vi "APLUS IEC 2015 Setup.vi"(0 "Remote IP Address":string="192.168.1.101", 1 "Instrument":string, 3 "Sample Rate (1: 0.25s)":u16(ring)=1 items=["0.1s", "0.25s", "0.5s", "1s", "2s", "5s"], 5 "Remote Port":u16=502, 7 "V Range (6: 600V)":u16(ring) items=["Auto", "15V", "30V", "60V", "150V", "300V", "600V"], 9 "A Range (12: 20A)":u16(ring) items=["Auto", "5mA", "10mA", "20mA", "50mA", "100mA", "200mA", "0.5A", "1A", "2A", "5A", "10A", "20A", "50mV", "100mV", "200mV", "2.5V", "5V", "10V"], 11 "error in":errorcluster, 13 "Reset WattHours":bool) -> (2 "VTHD":sgl format="%.3g", 6 "Header File":string[][](array[string]), 15 "error out":errorcluster)   [LabVIEW 2020]
uses:
  Type Definitions/APLUS Commands.ctl
  <vilib>/NI/Modbus Library/API/Wrapper/Create TCP Master.vi
  <vilib>/NI/Modbus Library/API/Master/Modbus Master.lvclass
  <vilib>/NI/Modbus Library/API/Wrapper/API Main.lvlib
panel:
  out "Date & Time":string
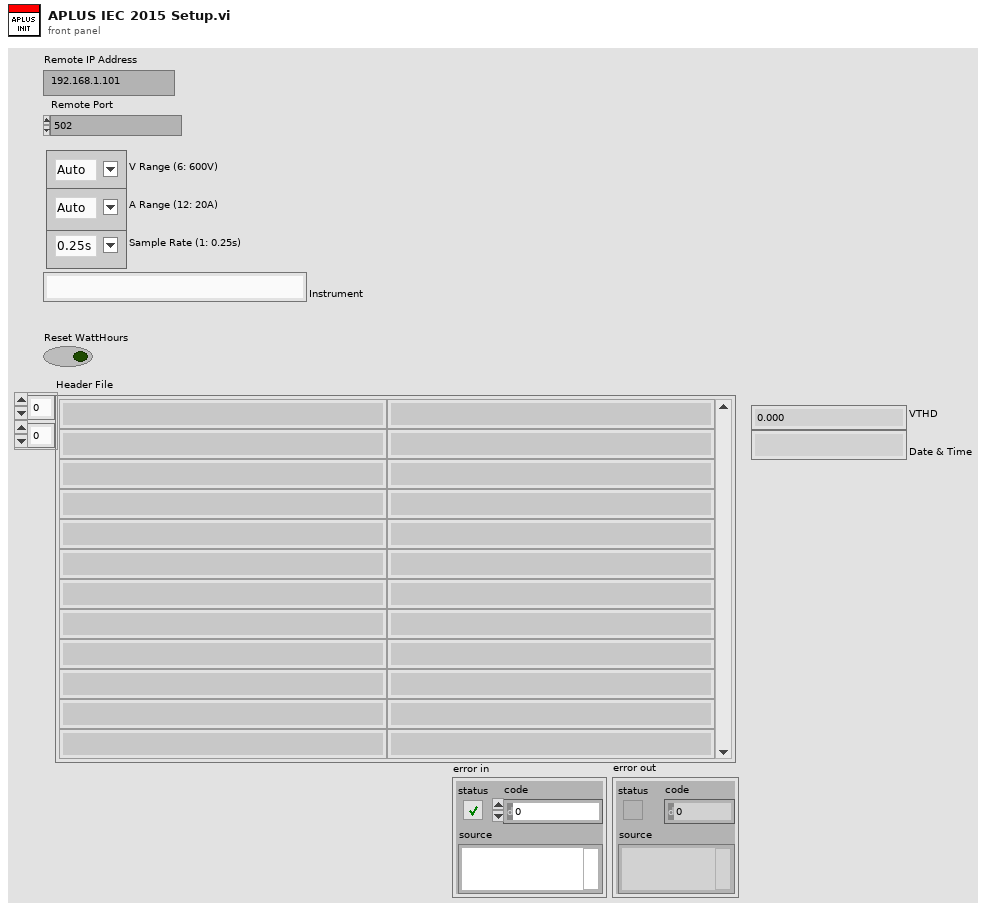
[diagram p1: front panel]
types:
  T1 = typedef "APLUS Commands.ctl" = u16
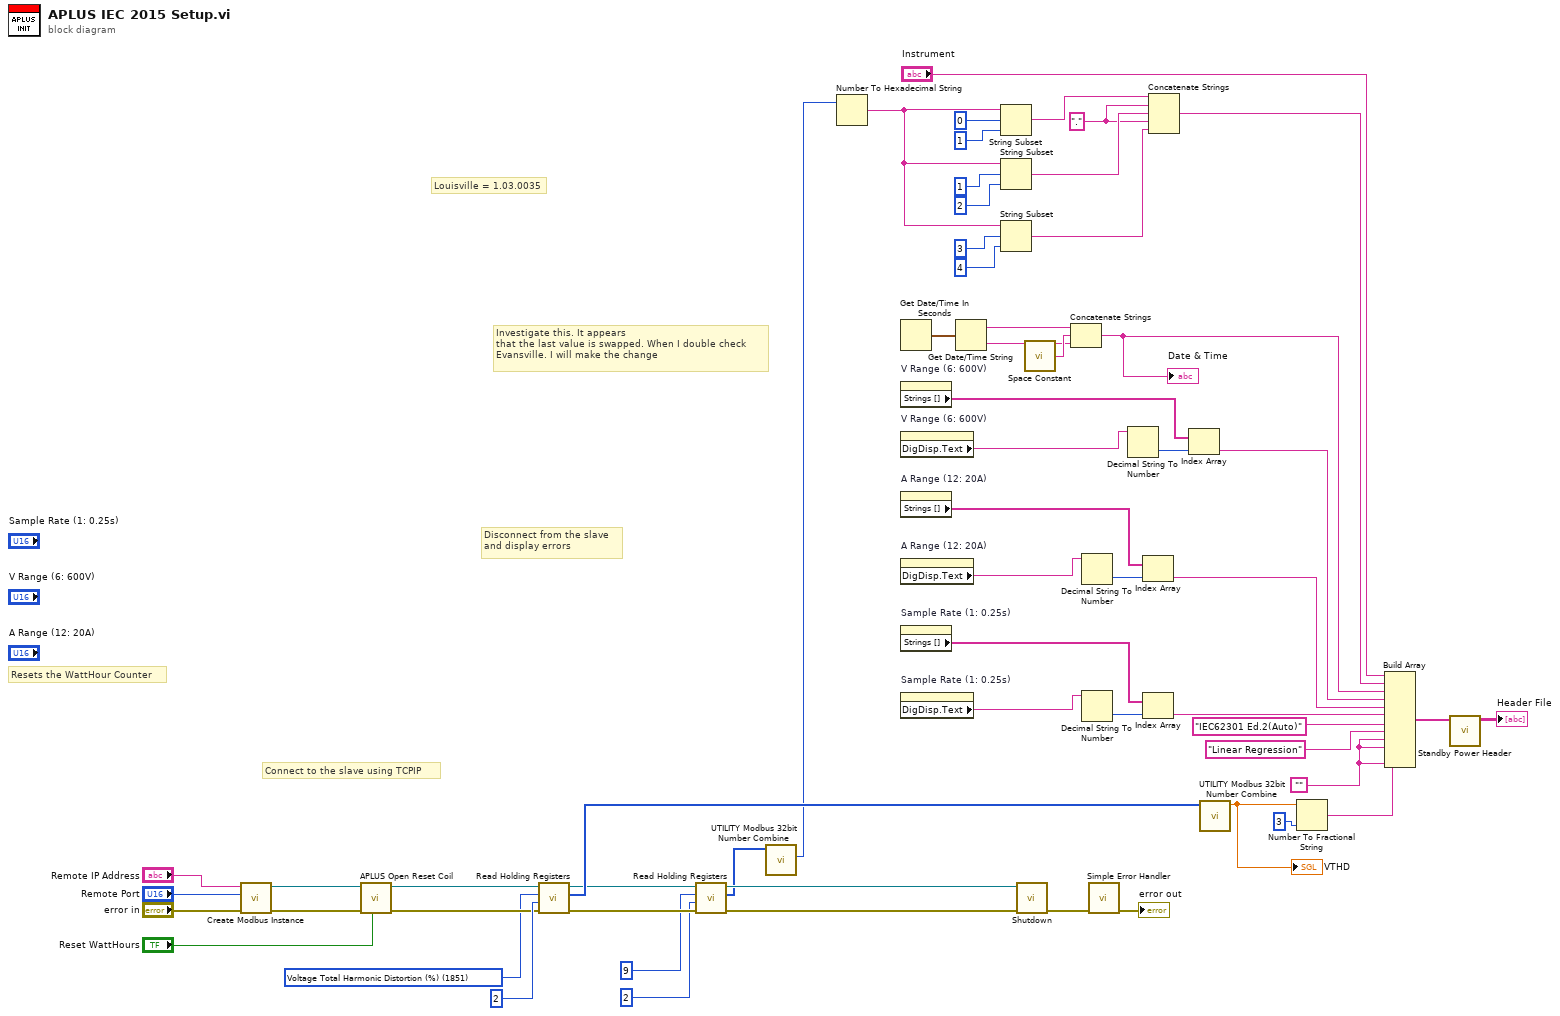
[diagram p0: block diagram]
diagram:
  w8 = "." ("string")
  w28 = T1 1851 items=["Voltage (V)"=1839, "RMS Current (Amps)"=1841, "Frequency (Hz)"=1843, "Power (Watts)"=1845, "Power Factor"=1847, "Apparent Power (VA)"=1849, "Voltage Total Harmonic Distortion (%)"=1851] ("APLUS Modbus Registers")
  w53 = ""
  # "Louisville = 1.03.0035"
  # "Investigate this. It appears\nthat the last value is swapped. When I double check\nEvansville. I will make the change"
  # "Resets the WattHour Counter"
  # "Disconnect from the slave\nand display errors"
  # "Connect to the slave using TCPIP"
  n1 = call-poly <vilib>:"Create Modbus Instance.vi"("error in"="error in", "port (502)"="Remote Port", "address"="Remote IP Address") -> ("error out"=w4:errorcluster, "TCP master instance"=w3:refnum<class "Modbus Master.lvclass">)  [unwired: 7 in]
  n2 = call "APLUS Open Reset Coil.vi"("Reset WattHours"="Reset WattHours", "error in (no error)"=w4, "Modbus Master in"=w3) -> ("error out"=w30:errorcluster, "Modbus Master out"=w29:refnum<class "Modbus Master.lvclass">)  [unwired: 7 in]
  n3 = call-dynamic "Read Holding Registers.vi"("error in"=w30, "number of inputs"=u16 2 ("Quantity"), "starting address"=w28, "Modbus master in"=w29) -> ("error out"=w23:errorcluster, "register values"=w50:u16[], "Modbus master out"=w25:refnum<class "Modbus Master.lvclass">)  [unwired: 5 in]
  n4 = call-dynamic "Read Holding Registers.vi"("error in"=w23, "number of inputs"=u16 2 ("Quantity"), "starting address"=u16 9, "Modbus master in"=w25) -> ("error out"=w22:errorcluster, "register values"=w19:u16[], "Modbus master out"=w24:refnum<class "Modbus Master.lvclass">)  [unwired: 5 in]
  n5 = call "UTILITY Modbus 32bit Number Combine.vi"("Holding Registers"=w19) -> ("word swapped"=w18:u32)  [unwired: 9 in, 1 out]
  n6 = Number To Hexadecimal String(2:w18) -> (0:w9:string)  [unwired: 1 in]
  n7 = Get Date/Time In Seconds() -> (seconds since 1Jan1904=w59:timestamp)
  n8 = property on="V Range (6: 600V)" class="Ring (strict)"() -> ("Strings []"=w37:string[])  [unwired: 2 in, 2 out]
  n9 = property on="V Range (6: 600V)" class="Ring (strict)"() -> ("DigDisp.Text"=w40:string)  [unwired: 2 in, 2 out]
  n10 = property on="A Range (12: 20A)" class="Ring (strict)"() -> ("Strings []"=w38:string[])  [unwired: 2 in, 2 out]
  n11 = property on="A Range (12: 20A)" class="Ring (strict)"() -> ("DigDisp.Text"=w39:string)  [unwired: 2 in, 2 out]
  n12 = property on="Sample Rate (1: 0.25s)" class="Ring (strict)"() -> ("Strings []"=w43:string[])  [unwired: 2 in, 2 out]
  n13 = property on="Sample Rate (1: 0.25s)" class="Ring (strict)"() -> ("DigDisp.Text"=w44:string)  [unwired: 2 in, 2 out]
  n14 = Get Date/Time String(seconds (now)=w59) -> (date string=w57:string, time string=w56:string)  [unwired: 2 in]
  n15 = String Subset(string=w9, offset (0)=0, length (rest)=1 ("length (rest)")) -> (substring=w15:string)
  n16 = String Subset(string=w9, offset (0)=1, length (rest)=2 ("length (rest)")) -> (substring=w12:string)
  n17 = String Subset(string=w9, offset (0)=3, length (rest)=4 ("length (rest)")) -> (substring=w7:string)
  n18 = call-dynamic "Shutdown.vi"("error in"=w22, "Modbus master in"=w24) -> ("error out"=w48:errorcluster)  [unwired: 9 in]
  n19 = call <vilib>:"Space Constant.vi"() -> ("String"=w58:string)
  n20 = Concatenate Strings(w57, w58, w56) -> (w46:string)
  "Date & Time" <- w46
  n21 = Decimal String To Number(string=w39) -> (number=w35:i32)  [unwired: 2 in, 1 out]
  n22 = Decimal String To Number(string=w44) -> (number=w42:i32)  [unwired: 2 in, 1 out]
  n23 = call <vilib>:"Simple Error Handler.vi"("error in (no error)"=w48) -> ("error out"=→"error out":errorcluster)  [unwired: 1 in, 7 out]
  n24 = Decimal String To Number(string=w40) -> (number=w36:i32)  [unwired: 2 in, 1 out]
  n25 = Index Array(array=w38, index=w35) -> (element=w33:string)
  n26 = Index Array(array=w43, index=w42) -> (element=w41:string)
  n27 = Concatenate Strings(w15, w8, w12, w8, w7) -> (w6:string)
  n28 = Index Array(array=w37, index=w36) -> (element=w34:string)
  n29 = call "UTILITY Modbus 32bit Number Combine.vi"("Holding Registers"=w50) -> ("Data"=w47:sgl)  [unwired: 9 in, 1 out]
  "VTHD" <- w47
  n30 = Number To Fractional String(number=w47, precision (6)=i16 3) -> (F-format string=w51:string)  [unwired: 2 in]
  n31 = Build Array("Instrument", w6, w46, w34, w33, w41, "IEC62301 Ed.2(Auto)" ("element"), "Linear Regression" ("element"), w53, w53, w51, w53) -> (w27:string[])
  n32 = call "Standby Power Header.vi"("Array"=w27) -> ("Header File"=→"Header File":string[][])  [unwired: 9 in, 1 out]
